vi "Write Voltage.vi"(8 "error in":errorcluster, 10 "Voltage":dbl, 11 "Acopian in":refnum<class "Acopian.lvclass">) -> (0 "error out":errorcluster, 3 "Acopian out":refnum<class "Acopian.lvclass">)   [LabVIEW 2019, in "Acopian.lvlib" / "Acopian.lvclass"]
uses:
  Library/Acopian.lvclass
  builds/Instruments/PowerSupply.lvlibp/Library/PowerSupply.lvclass
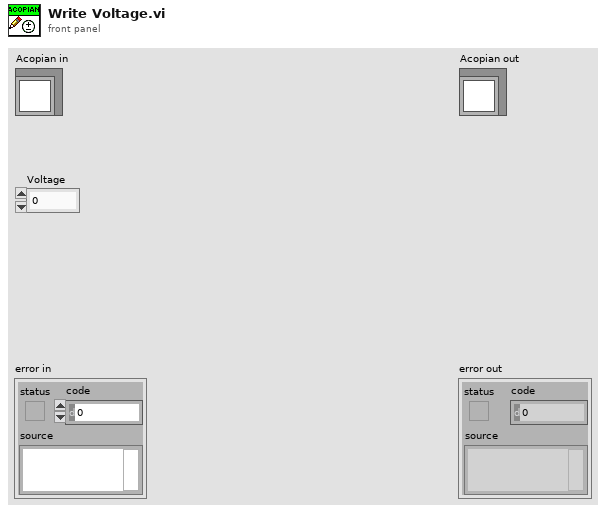
[diagram p1: front panel]
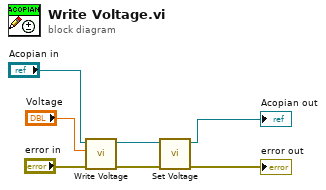
[diagram p0: block diagram]
diagram:
  n1 = call-parent "Write Voltage.vi"("error in"="error in", "Voltage"="Voltage", "PowerSupply in"="Acopian in") -> ("error out"=w3:errorcluster, "PowerSupply out"=w4:refnum<class "Acopian.lvclass">)  [unwired: 7 in]
  n2 = call "Set Voltage.vi"("error in"=w3, "Acopian in"=w4) -> ("error out"=→"error out":errorcluster, "Acopian out"=→"Acopian out":refnum<class "Acopian.lvclass">)  [unwired: 8 in]
